vi "Read Digital Channel.vi"(8 "error in":errorcluster, 11 "digital channel in":refnum<class "Digital Channel.lvclass">) -> (0 "error out":errorcluster, 1 "default value":bool, 2 "name":string, 3 "digital channel out":refnum<class "Digital Channel.lvclass">, 4 "index":i32)   [LabVIEW 2017, in "Scan Engine Scripting.lvlib" / "Digital Channel.lvclass"]
doc: "Reads the name, index and type of a channel."
uses:
  Digital Channel.lvclass
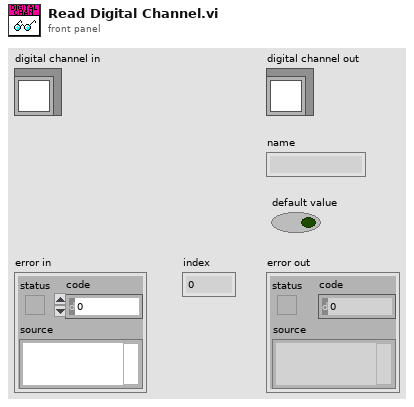
[diagram p1: front panel]
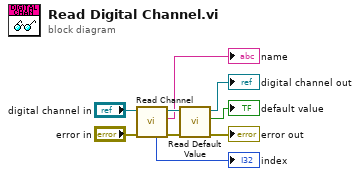
[diagram p0: block diagram]
diagram:
  n1 = call-dynamic "Read Channel.vi"("error in (no error)"="error in", "Channel in"="digital channel in") -> ("error out"=w4:errorcluster, "name"=→"name":string, "Channel out"=w7:refnum<class "Digital Channel.lvclass">, "index"=→"index":i32)  [unwired: 4 in, 2 out]
  n2 = call-dynamic "Read Default Value.vi"("error in"=w4, "digital channel in"=w7) -> ("error out"=→"error out":errorcluster, "default value"=→"default value":bool, "digital channel out"=→"digital channel out":refnum<class "Digital Channel.lvclass">)  [unwired: 7 in]
